vi "FGV-GlobalEventRef.vi"(6 "Create(F)":bool, 8 "error in (no error)":errorcluster) -> (0 "error out":errorcluster, 3 "JKISM Global Log Event":refnum<user-event>)   [LabVIEW 2014, in "JKI State Machine++.lvlib"]
uses:
  JKI State Machine++.lvlib
  Typedef/_JKISM Current State.ctl
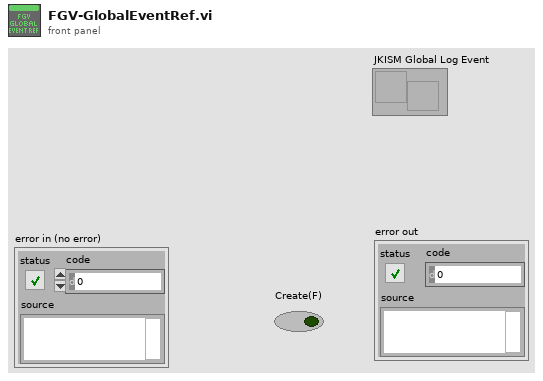
[diagram p1: front panel]
types:
  T1 = typedef "JKI State Machine++.lvlib/_JKISM Current State.ctl" = cluster{"Name(\"\" to use uuid)":string, "Current State":string, "Arguments":string, "Argument - State":string, "From Who":string, "Complete(T)/Start(F)":bool}
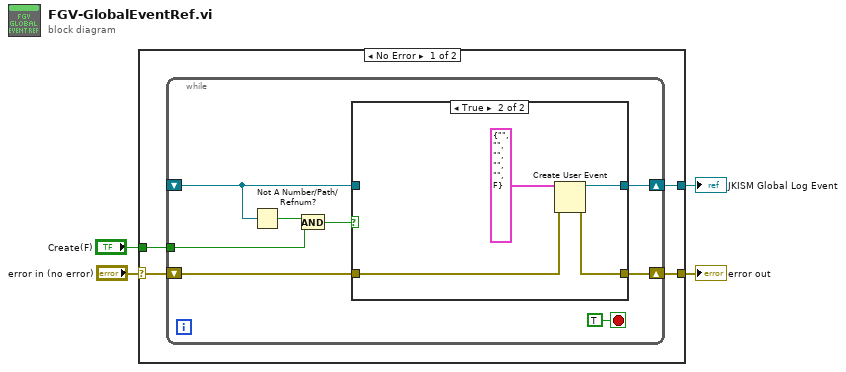
[diagram p0: block diagram]
diagram:
  n1 = case shown="No Error" "error in (no error)" {
    selector: "error in (no error)" -> [w7 w23]
    tunnel: [w8 _] -> w4
    tunnel: [w6 w23] -> w2
    tunnel: "Create(F)" -> [w5 _]
    frame No Error {
      n2 = while {
        shift-right: [w14] -> w6
        shift-left: w7 -> [w15]
        shift-right: [w16] -> w8
        shift-left: _ -> [w12]
        tunnel: w5 -> [w9]
        stop <- TRUE stop-if-true
        n3 = Not A Number/Path/Refnum?(number/path/refnum=w12) -> (NaN/Path/Refnum?=w10:bool)
        n4 = And(x=w10, y=w9) -> (x .and. y?=w11:bool)
        n5 = case shown="True" w11 {
          tunnel: [w18 w21] -> w16
          tunnel: w15 -> [w17 w20]
          tunnel: [w17 w19] -> w14
          tunnel: w12 -> [w18 _]
          frame False {
          }
          frame True {
            n6 = Create User Event(user event datatype=T1 {"Name(\"\" to use uuid)"="", "Current State"="", "Arguments"="", "Argument - State"="", "From Who"="", "Complete(T)/Start(F)"=FALSE} ("Cross JKI State Machine Data"), error in=w20) -> (user event=w21:refnum<user-event>, error out=w19:errorcluster)
          }
        }
      }
    }
    frame Error {
    }
  }
  "JKISM Global Log Event" <- w4
  "error out" <- w2
